vi "RunProbeCycle.vi"(1 "SweepInfo":T1={"Current Range"=1e-10, "Source Measure Unit Channel (0: Channel A)"=0, "Waveform"={"t0"=timestamp(0 s since 1904-01-01), "dt"=1.0, "Y"=[]}, "VISA resource name"="", "CodeText"=""}, 2 "Lift Distance (um)":dbl, 5 "ScaleTranslation":T2, 6 "Status":refnum<vi>, 7 "PlayButton":refnum<k24>, 8 "FileInfo":T3={"Die"="", "Wafer"="", "Path"=path "", "url"="https://raxdatastore.azurewebsites.net/api/DataUploadJson?code=aWWmuAqIJVgQhV7ha3pemybWHXVmpxXI7auinBch5Z66k9y4fpn1vQ==&Tags="}, 9 "Microsites":refnum<k24>, 10 "XYGraph in":refnum<vi>) -> (0 "Fit":dbl[][](array[numeric]))   [LabVIEW 2020]
uses:
  C:/Projects/RaxTagServer/LabviewDXFViewer/LabviewDXFViewer/bin/Release/LabviewDXFViewer.exe
  LabviewDXFViewer/bin/Release/LabviewDXFViewer.exe
  System.Drawing
  <vilib>/Utility/file.llb/Write Delimited Spreadsheet (string).vi
panel:
  out "error out 2":errorcluster
  out "Junction Name":string
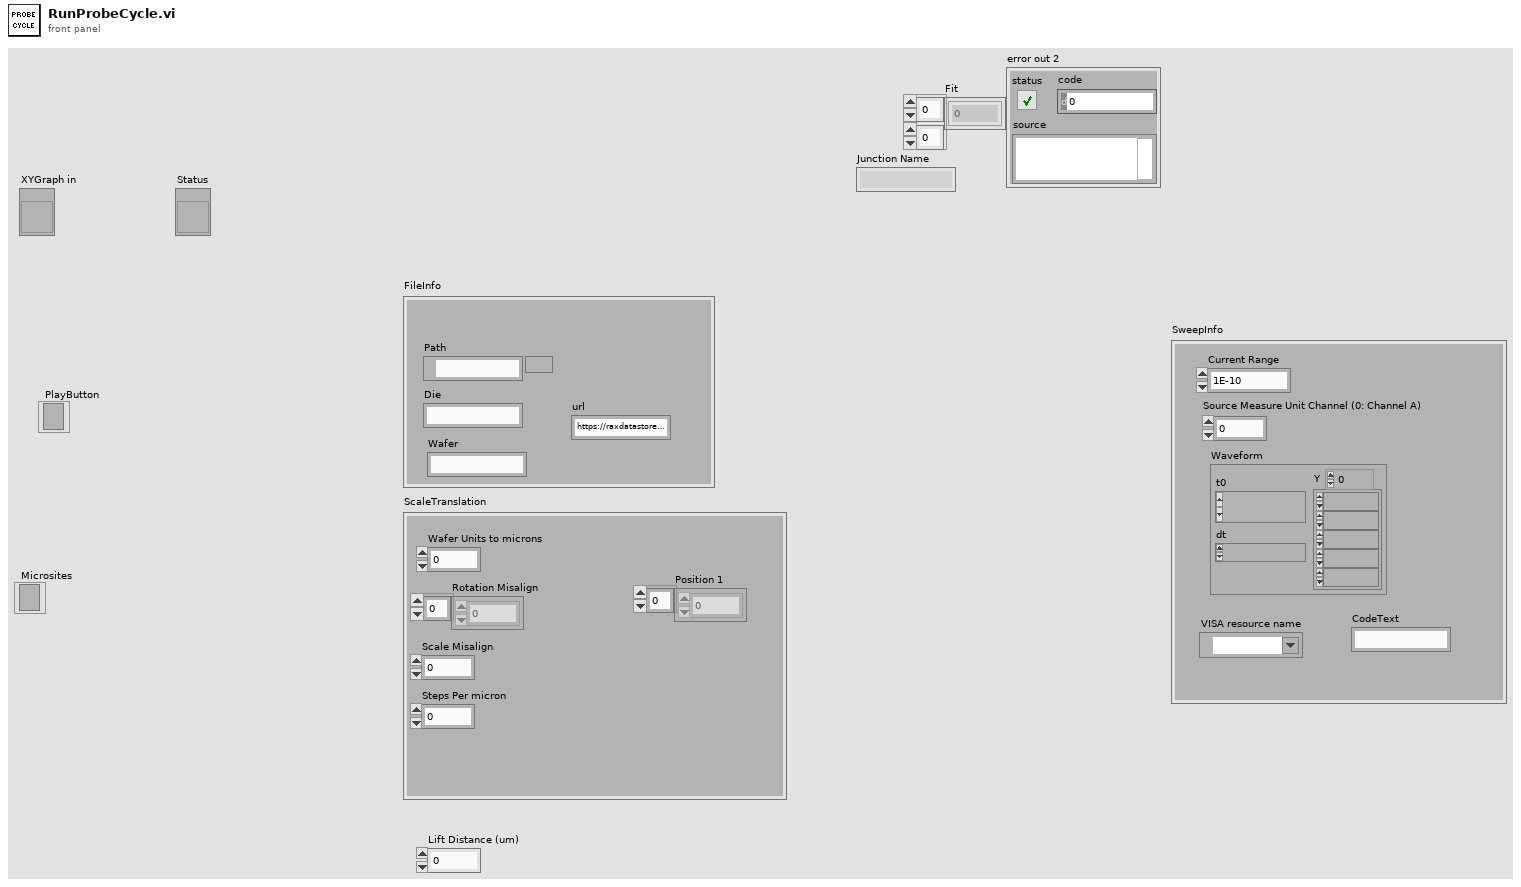
[diagram p1: front panel]
types:
  T1 = cluster{"Current Range":dbl, "Source Measure Unit Channel (0: Channel A)":i32, "Waveform":waveform(dbl), "VISA resource name":refnum<visa-resource-name>, "CodeText":string}
  T2 = cluster{"Wafer Units to microns":dbl, "Rotation Misalign":dbl[], "Scale Misalign":dbl, "Steps Per micron":dbl, "Position 1":i32[]}
  T3 = cluster{"Die":string, "Wafer":string, "Path":path, "url":string}
  T4 = cluster{"Coordinates":dbl[], "Junction Name":string, "Orientation":string}
  T5 = enum16{"Left Button", "Center Button", "Right Button", "Window Close"}
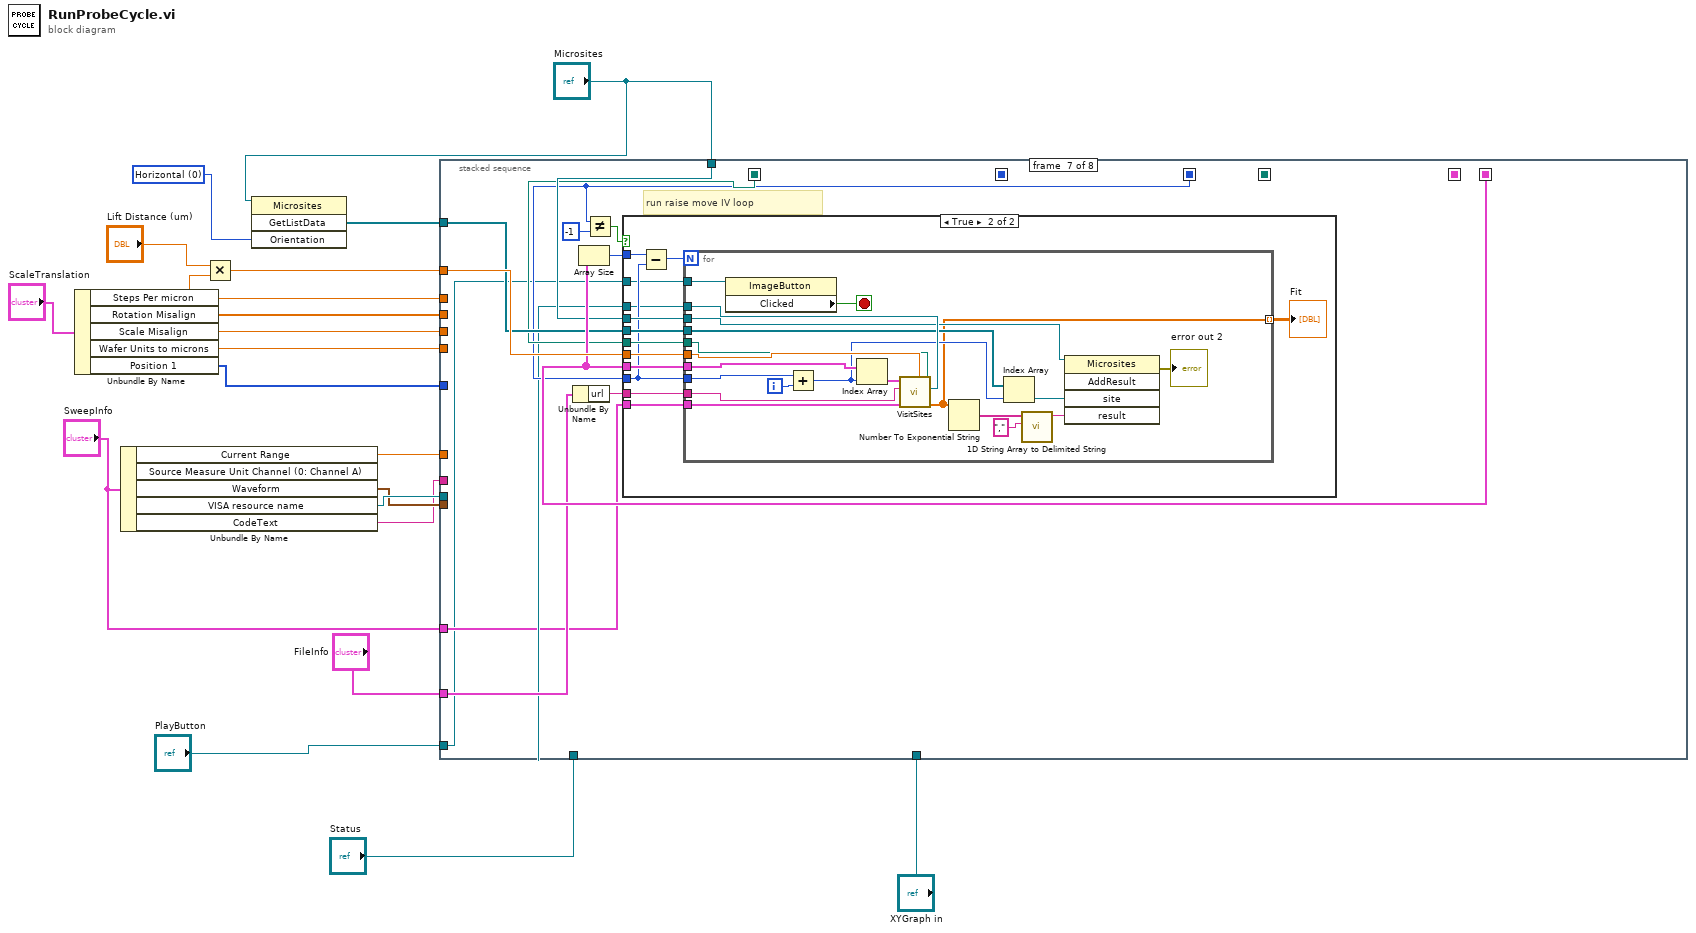
[diagram p0: block diagram]
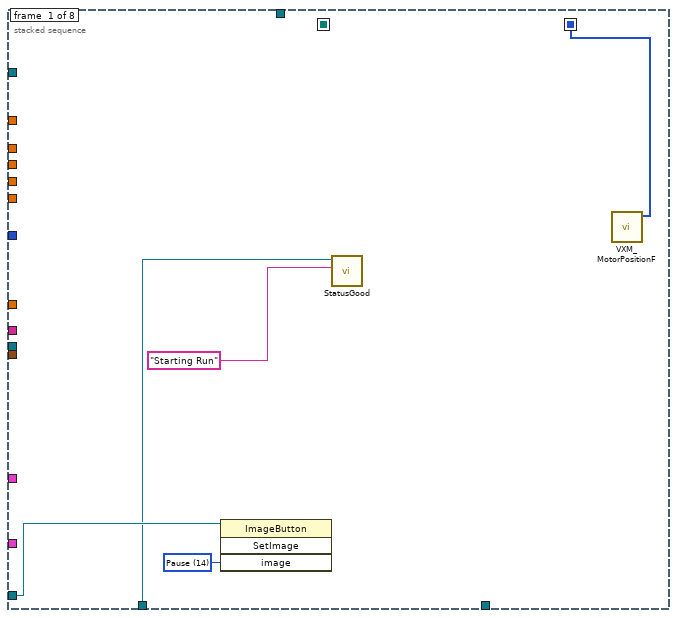
[diagram p2: hidden frame]
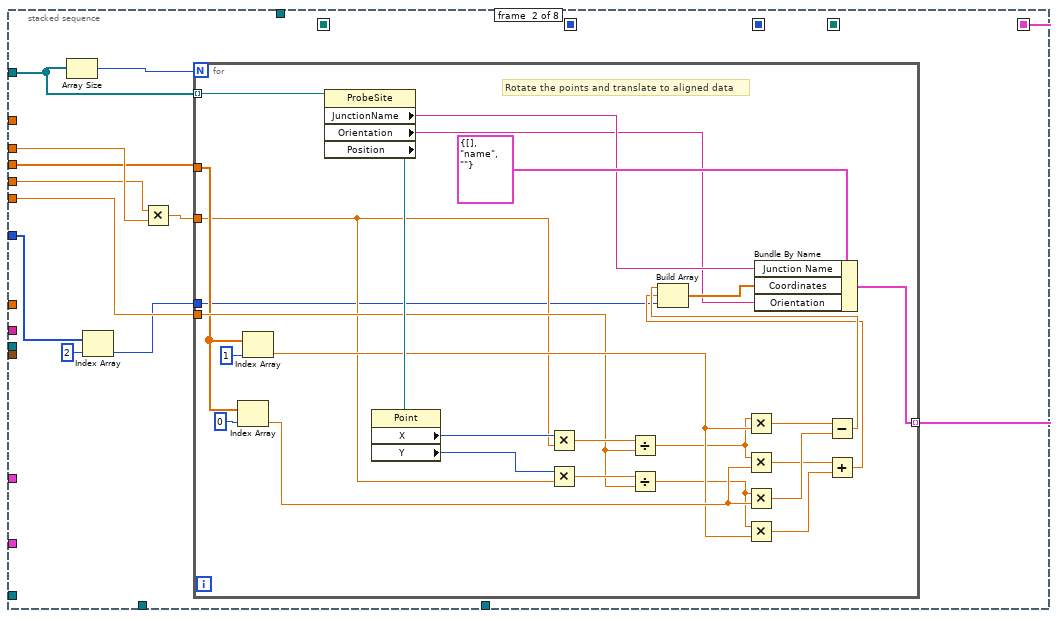
[diagram p3: hidden frame]
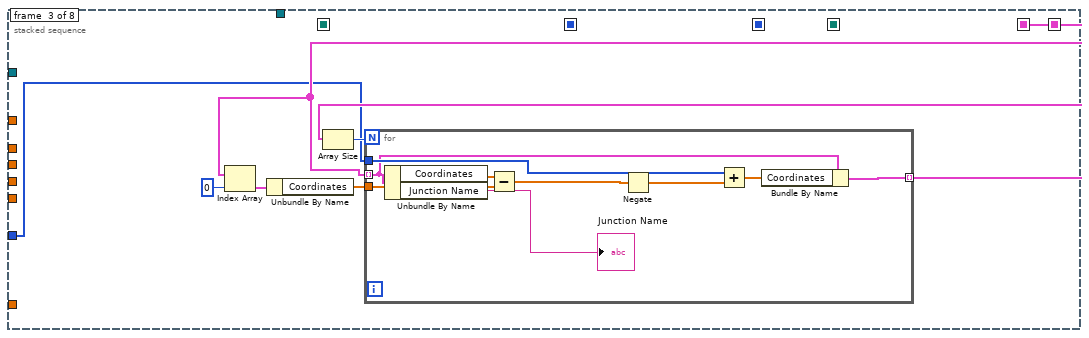
[diagram p4: hidden frame]
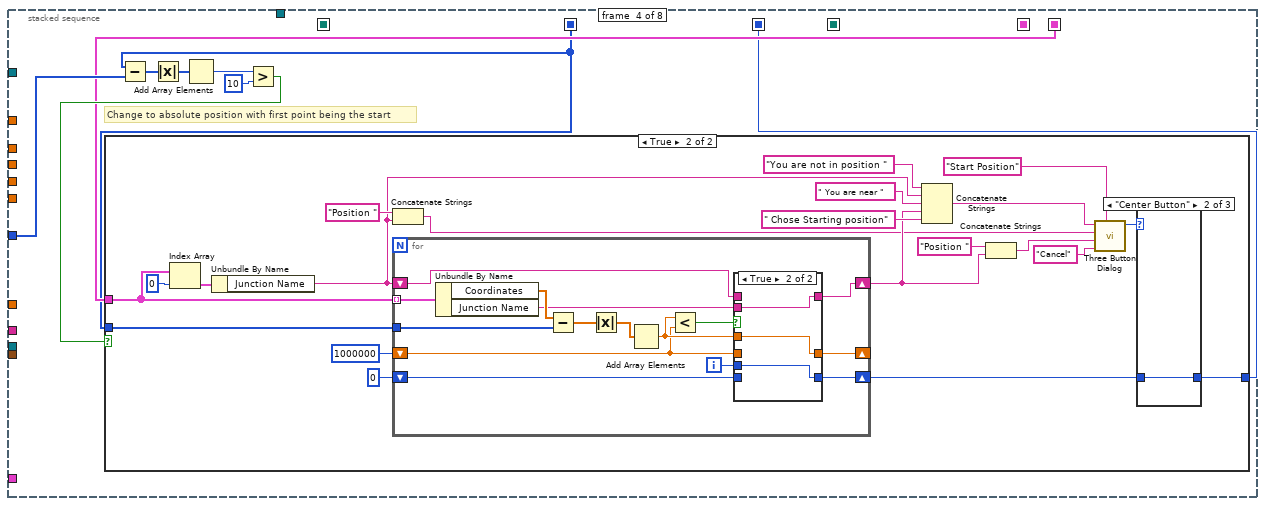
[diagram p5: hidden frame]
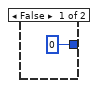
[diagram p6: hidden frame]
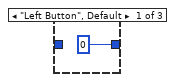
[diagram p8: hidden frame]
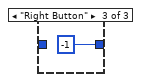
[diagram p9: hidden frame]
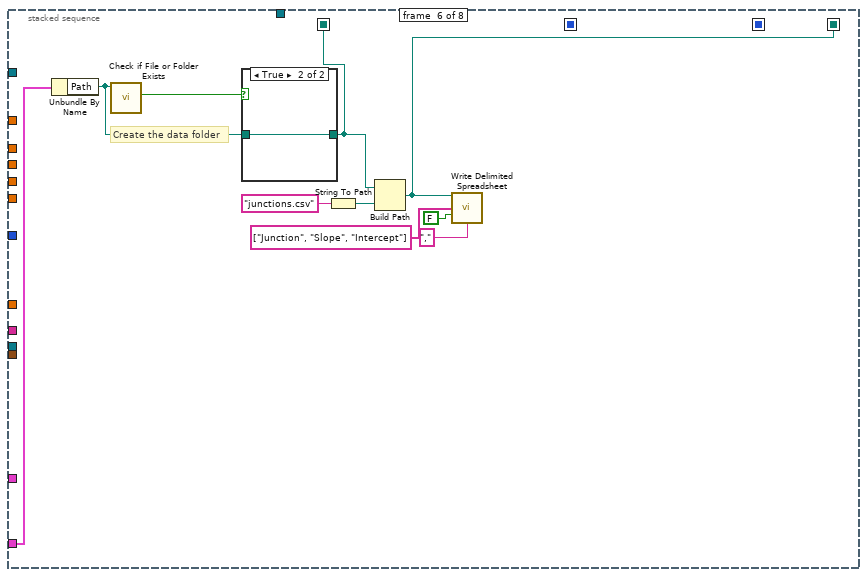
[diagram p11: hidden frame]
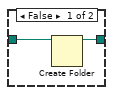
[diagram p12: hidden frame]
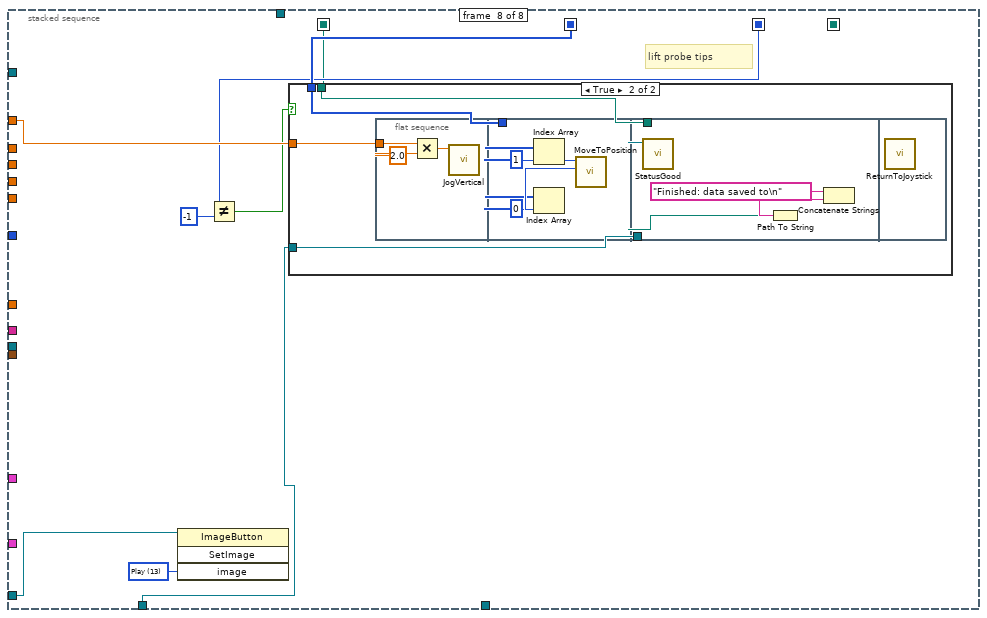
[diagram p14: hidden frame]
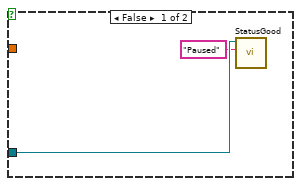
[diagram p15: hidden frame]
diagram:
  w7 = 0 items=["Horizontal", "Vertical"] ("Orientation")
  n1 = Unbundle By Name("ScaleTranslation") -> ("Steps Per micron"=w16:dbl, "Rotation Misalign"=w14:dbl[], "Scale Misalign"=w15:dbl, "Wafer Units to microns"=w13:dbl, "Position 1"=w5:i32[])
  n2 = Unbundle By Name("SweepInfo") -> ("Current Range"=w12:dbl, "Waveform"=w10:waveform(dbl), "VISA resource name"=w11:refnum<visa-resource-name>, "CodeText"=w6:string)  [unwired: 1 out]
  n3 = Multiply(x="Lift Distance (um)", y=w16) -> (x*y=w20:dbl)
  n4 = invoke class="Microsites" method="GetListData"(reference="Microsites", "Orientation"=w7) -> ("GetListData"=w8:refnum<k24>[])  [unwired: 2 in, 3 out]
  n5 = stacked-sequence {
    seq-local: [_ w32 _ _ _ _ _ _] -> [_ _ w66 _ _ _ _ _]
    seq-local: [w25 _ _ _ _ _ _ _] -> [_ _ _ w80 _ _ _ w202]
    seq-local: [_ _ w65 _ _ _ _ _] -> [_ _ _ w82 _ _ w160 _]
    seq-local: [_ _ _ _ _ w137 _ _] -> [_ _ _ _ _ _ w155 w196]
    seq-local: [_ _ _ w81 _ _ _ _] -> [_ _ _ _ _ _ w153 w200]
    seq-local: [_ _ _ _ _ w135 _ _] -> [_ _ _ _ _ _ _ _]
    tunnel: w10 -> [_ _ _ _ _ _ _ _]
    tunnel: w20 -> [_ _ _ _ _ _ w161 w203]
    tunnel: w16 -> [_ w36 _ _ _ _ _ _]
    tunnel: w6 -> [_ _ _ _ _ _ _ _]
    tunnel: "Microsites" -> [_ _ _ _ _ _ w159 _]
    tunnel: w8 -> [_ w33 _ _ _ _ w158 _]
    tunnel: w12 -> [_ _ _ _ _ _ _ _]
    tunnel: "FileInfo" -> [_ _ _ _ _ w138 w157 _]
    tunnel: w15 -> [_ w31 _ _ _ _ _ _]
    tunnel: w14 -> [_ w30 _ _ _ _ _ _]
    tunnel: w13 -> [_ w29 _ _ _ _ _ _]
    tunnel: w11 -> [_ _ _ _ _ _ _ _]
    tunnel: w5 -> [_ w28 w64 w83 _ _ _ _]
    tunnel: "XYGraph in" -> [_ _ _ _ _ _ w150 _]
    tunnel: "SweepInfo" -> [_ _ _ _ _ _ w149 _]
    tunnel: "PlayButton" -> [w24 _ _ _ _ _ w148 w198]
    tunnel: "Status" -> [w21 _ _ _ _ _ _ w195]
    frame #0 {
      w23 = 14 items=["Left", "LeftBig", "LeftSmall", "Right", "RightBig", "RightSmall", "Up", "UpBig", "UpSmall", "Down", "DownBig", "DownSmall", "Zero", "Play", "Pause", "Load", "Lower", "Raise", "Home", "Home2"] ("image")
      n6 = invoke class="ImageButton" method="SetImage"(reference=w24, "image"=w23) -> ()  [unwired: 2 in, 4 out]
      n7 = call "StatusGood.vi"("Text.Text"="Starting Run" ("Run Message"), "String in"=w21) -> ()  [unwired: 10 in]
      n8 = call "VXM_MotorPositionF.vi"() -> ("Position"=w25:i32[])  [unwired: 11 in]
    }
    frame #1 {
      n9 = Array Size(array=w33) -> (size(s)=w34:i32)
      n10 = Index Array(array=w28, index=2) -> (element=w26:i32)
      n11 = Multiply(x=w31, y=w36) -> (x*y=w35:dbl)
      n12 = for {
        N: w34 -> [_]
        tunnel: w33 -> [w62] mode=indexing
        tunnel: [w45] -> w32 mode=indexing
        tunnel: w29 -> [w40]
        tunnel: w30 -> [w39]
        tunnel: w35 -> [w38]
        tunnel: w26 -> [w37]
        # "Rotate the points and translate to aligned data"
        n13 = Index Array(array=w39, index=0) -> (element=w55:dbl)
        n14 = Index Array(array=w39, index=1) -> (element=w54:dbl)
        n15 = property class="ProbeSite"(reference=w62) -> ("JunctionName"=w47:string, "Orientation"=w46:string, "Position"=w63:refnum<k24>)  [unwired: 1 in, 2 out]
        n16 = property class="Point"(reference=w63) -> ("X"=w61:i32, "Y"=w60:i32)  [unwired: 1 in, 2 out]
        n17 = Multiply(x=w61, y=w38) -> (x*y=w43:dbl)
        n18 = Multiply(x=w60, y=w38) -> (x*y=w41:dbl)
        n19 = Divide(x=w43, y=w40) -> (x/y=w44:dbl)
        n20 = Divide(x=w41, y=w40) -> (x/y=w42:dbl)
        n21 = Multiply(x=w44, y=w54) -> (x*y=w57:dbl)
        n22 = Multiply(x=w44, y=w55) -> (x*y=w53:dbl)
        n23 = Multiply(x=w42, y=w55) -> (x*y=w56:dbl)
        n24 = Multiply(x=w42, y=w54) -> (x*y=w52:dbl)
        n25 = Subtract(x=w57, y=w56) -> (x-y=w51:dbl)
        n26 = Add(x=w53, y=w52) -> (x+y=w50:dbl)
        n27 = Build Array(w51, w50, w37) -> (w49:dbl[])
        n28 = Bundle By Name(cluster=T4 {"Coordinates"=[], "Junction Name"="name", "Orientation"=""} ("input cluster"), "Junction Name"=w47, "Coordinates"=w49, "Orientation"=w46) -> (w45:T4)
      }
    }
    frame #2 {
      n29 = Index Array(array=w66, index=0) -> (element=w68:T4)
      n30 = Unbundle By Name(w68) -> ("Coordinates"=w67:dbl[])
      n31 = Array Size(array=w66) -> (size(s)=w69:i32)
      n32 = for {
        N: w69 -> [_]
        tunnel: w64 -> [w77]
        tunnel: w67 -> [w78]
        tunnel: w66 -> [w76] mode=indexing
        tunnel: [w74] -> w65 mode=indexing
        n33 = Unbundle By Name(w76) -> ("Coordinates"=w79:dbl[], "Junction Name"=→"Junction Name":string)
        n34 = Subtract(x=w79, y=w78) -> (x-y=w73:dbl[])
        n35 = Negate(x=w73) -> (-x=w71:dbl[])
        n36 = Add(x=w77, y=w71) -> (x+y=w75:dbl[])
        n37 = Bundle By Name(cluster=w76, "Coordinates"=w75) -> (w74:T4)
      }
    }
    frame #3 {
      # "Change to absolute position with first point being the start"
      n38 = Subtract(x=w80, y=w83) -> (x-y=w88:i32[])
      n39 = Absolute Value(x=w88) -> (abs(x)=w87:i32[])
      n40 = Add Array Elements(numeric array=w87) -> (sum=w86:i32)
      n41 = Greater?(x=w86, y=10) -> (0:w84:bool)
      n42 = case shown="True" w84 {
        tunnel: [0 w103] -> w81
        tunnel: w82 -> [_ w99]
        tunnel: w80 -> [_ w90]
        frame False {
        }
        frame True {
          n43 = Index Array(array=w99, index=0) -> (element=w109:T4)
          n44 = Unbundle By Name(w109) -> ("Junction Name"=w92:string)
          n45 = Concatenate Strings("Position " ("Left Button Text (\"Yes\")"), w92) -> (w93:string)
          n46 = for {
            tunnel: w99 -> [w123] mode=indexing
            tunnel: w90 -> [w121]
            shift-right: [w115] -> w97
            shift-left: 0 -> [w114]
            shift-right: [w116] -> w96
            shift-left: w92 -> [w117]
            shift-right: [w113] -> _
            shift-left: 1000000 -> [w111]
            i -> [w118]
            n47 = Unbundle By Name(w123) -> ("Coordinates"=w122:dbl[], "Junction Name"=w120:string)
            n48 = Subtract(x=w122, y=w121) -> (x-y=w125:dbl[])
            n49 = Absolute Value(x=w125) -> (abs(x)=w124:dbl[])
            n50 = Add Array Elements(numeric array=w124) -> (sum=w112:dbl)
            n51 = Less?(x=w112, y=w111) -> (x < y?=w119:bool)
            n52 = case shown="True" w119 {
              tunnel: w120 -> [_ w131]
              tunnel: w117 -> [w128 _]
              tunnel: [w128 w131] -> w116
              tunnel: w118 -> [_ w130]
              tunnel: [w127 w130] -> w115
              tunnel: w114 -> [w127 _]
              tunnel: w111 -> [w126 _]
              tunnel: [w126 w129] -> w113
              tunnel: w112 -> [_ w129]
              frame False {
              }
              frame True {
              }
            }
          }
          n53 = Concatenate Strings("You are not in position " ("message"), w92, " You are near " ("string"), w96, " Chose Starting position" ("string")) -> (w106:string)
          n54 = Concatenate Strings("Position " ("string"), w96) -> (w105:string)
          n55 = call <vilib>:"Three Button Dialog.vi"("Window Title (\"\")"="Start Position" ("Window Title (\"\")"), "Right Button Text (\"Cancel\")"="Cancel" ("Right Button Text (\"Cancel\")"), "Center Button Text (\"No\")"=w105, "Left Button Text (\"Yes\")"=w93, "message"=w106) -> ("Which Button?"=w102:T5)  [unwired: 6 in]
          n56 = case shown="\"Center Button\"" w102 {
            tunnel: [0 w133 -1] -> w103
            tunnel: w97 -> [_ w133 _]
            frame "Left Button", Default {
            }
            frame "Center Button" {
            }
            frame "Right Button" {
            }
          }
        }
      }
    }
    frame #4 {
      # "Program Keithley"
    }
    frame #5 {
      # "Create the data folder"
      n57 = Unbundle By Name(w138) -> ("Path"=w136:path)
      n58 = call <vilib>:"Check if File or Folder Exists.vi"("path"=w136) -> ("file or folder exists?"=w144:bool)  [unwired: 8 in, 2 out]
      n59 = case shown="True" w144 {
        tunnel: w136 -> [w146 w147]
        tunnel: [w145 w147] -> w137
        frame False {
          n60 = Create Folder(path (use dialog)=w146) -> (created path=w145:path)  [unwired: 2 in, 2 out]
        }
        frame True {
        }
      }
      n61 = String To Path(string="junctions.csv") -> (path=w143:path)
      n62 = Build Path(base path=w137, name or relative path=w143) -> (appended path=w135:path)
      n63 = call-poly <vilib>:"Write Delimited Spreadsheet.vi"("file path (dialog if empty)"=w135, "1D data"=string[] ["Junction", "Slope", "Intercept"], "append to file? (new file:F)"=FALSE, "delimiter (\\t)"="," ("delimiter (\\t)")) -> ()  [unwired: 10 in, 2 out]
    }
    frame #6 {
      # "run raise move IV loop"
      n64 = Unbundle By Name(w157) -> ("url"=w156:string)
      n65 = Array Size(array=w160) -> (size(s)=w154:i32)
      n66 = Not Equal?(x=w153, y=-1) -> (x != y?=w152:bool)
      n67 = case shown="True" w152 {
        tunnel: w161 -> [_ w174]
        tunnel: w160 -> [_ w173]
        tunnel: w159 -> [_ w171]
        tunnel: w158 -> [_ w170]
        tunnel: w156 -> [_ w169]
        tunnel: w155 -> [_ w168]
        tunnel: w153 -> [_ w165]
        tunnel: w154 -> [_ w166]
        tunnel: w150 -> [_ w164]
        tunnel: w149 -> [_ w163]
        tunnel: w148 -> [_ w162]
        frame False {
        }
        frame True {
          n68 = Subtract(x=w166, y=w165) -> (x-y=w167:i32)
          n69 = for {
            N: w167 -> [_]
            tunnel: w164 -> [w193]
            tunnel: w174 -> [w194]
            tunnel: [w182] -> w172 mode=indexing
            tunnel: w173 -> [w192]
            tunnel: w171 -> [w191]
            tunnel: w170 -> [w190]
            tunnel: w169 -> [w187]
            tunnel: w168 -> [w186]
            tunnel: w165 -> [w185]
            tunnel: w163 -> [w177]
            tunnel: w162 -> [w176]
            i -> [w189]
            stop <- w175 stop-if-true
            n70 = property class="ImageButton"(reference=w176) -> ("Clicked"=w175:bool)  [unwired: 1 in, 2 out]
            n71 = Add(x=w185, y=w189) -> (x+y=w183:i32)
            n72 = Index Array(array=w192, index=w183) -> (element=w184:T4)
            n73 = call "VisitSites.vi"("Microsite"=w184, "url"=w187, "SweepInfo"=w177, "Lift Distance (steps)"=w194, "Path"=w186, "XYGraph Refnum"=w193) -> ("Fit"=w182:dbl[])  [unwired: 4 in]
            n74 = Number To Exponential String(number=w182) -> (E-format string=w181:string[])  [unwired: 3 in]
            n75 = Index Array(array=w190, index=w183) -> (element=w188:refnum<k24>)
            n76 = call <vilib>:"1D String Array to Delimited String.vi"("delimiter"=",", "string array"=w181) -> ("delimited string"=w179:string)  [unwired: 9 in]
            n77 = invoke class="Microsites" method="AddResult"(reference=w191, "site"=w188, "result"=w179) -> (error out=→"error out 2":errorcluster)  [unwired: 2 in, 4 out]
          }
          "Fit" <- w172
        }
      }
    }
    frame #7 {
      w197 = 13 items=["Left", "LeftBig", "LeftSmall", "Right", "RightBig", "RightSmall", "Up", "UpBig", "UpSmall", "Down", "DownBig", "DownSmall", "Zero", "Play", "Pause", "Load", "Lower", "Raise", "Home", "Home2"] ("image")
      # "lift probe tips"
      n78 = invoke class="ImageButton" method="SetImage"(reference=w198, "image"=w197) -> ()  [unwired: 2 in, 4 out]
      n79 = Not Equal?(x=w200, y=-1) -> (x != y?=w199:bool)
      n80 = case shown="True" w199 {
        tunnel: w203 -> [_ w209]
        tunnel: w202 -> [_ w208]
        tunnel: w196 -> [_ w207]
        tunnel: w195 -> [w205 w206]
        frame False {
          n81 = call "StatusGood.vi"("Text.Text"="Paused", "String in"=w205) -> ()  [unwired: 10 in]
        }
        frame True {
          n82 = flat-sequence {
            tunnel: w209 -> [w212]
            tunnel: w208 -> [w215]
            tunnel: w207 -> [w220]
            tunnel: w206 -> [w218]
            frame #0 {
              n83 = Multiply(x=w212, y=2.0) -> (x*y=w210:dbl)
              n84 = call "JogVertical.vi"("Numeric"=w210) -> ()  [unwired: 11 in]
            }
            frame #1 {
              n85 = Index Array(array=w215, index=1) -> (element=w217:i32)
              n86 = Index Array(array=w215, index=0) -> (element=w216:i32)
              n87 = call "MoveToPosition.vi"("Y"=w216, "X"=w217) -> ()  [unwired: 10 in]
            }
            frame #2 {
              n88 = call "StatusGood.vi"("String in"=w218) -> ()  [unwired: 11 in]
              n89 = Path To String(path=w220) -> (string=w221:string)
              n90 = Concatenate Strings("Finished: data saved to\n" ("Text.Text"), w221) -> ()  [unwired: 1 out]
            }
            frame #3 {
              n91 = call "ReturnToJoystick.vi"() -> ()  [unwired: 12 in]
            }
          }
        }
      }
    }
  }
